vi "Router.vi"(8 "error in (no error)":errorcluster, 11 "Node Ptr":T1 format="%.0x") -> (0 "error out":errorcluster)   [LabVIEW 2016, in "PXImc Custom Device System Explorer.lvlib"]
uses:
  PXImc Custom Device System Explorer.lvlib
  <vilib>/NI Veristand/Custom Device API/Custom Device Item Ref.ctl
  Shared/Constants.vi
  <vilib>/NI Veristand/Custom Device API/Get Item Property (Variant).vi
  <vilib>/NI Veristand/Custom Device API/Set Item Property (Variant).vi
  <vilib>/NI VeriStand/Custom Device API/Custom Device API.lvlib
  Shared/PXImc Custom Device Shared.lvlib
panel:
  out "PXImc Resource Names":string[](array[string])
  in  "Connection Timeout (s)":dbl
  in  "Readers Buffer Size":u64
  in  "Configution Files Path":path
  in  "Load Configuration":bool
  in  "Header":cluster{"Section Name":string}={"Section Name"="Custom Device Item Settings"}
  in  "Description":string
  in  "Name":string
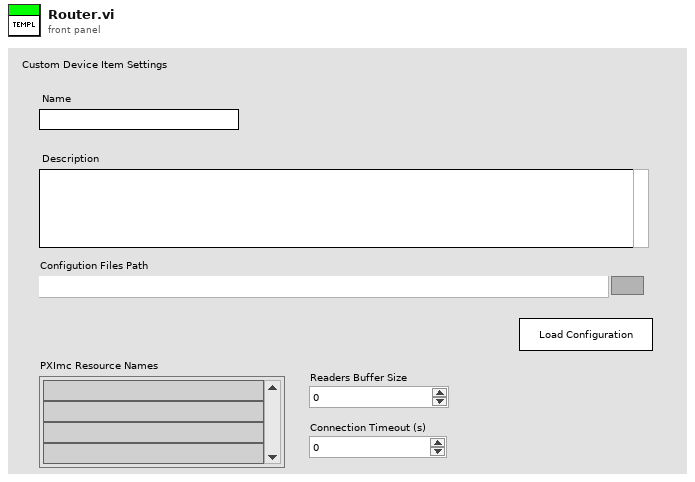
[diagram p1: front panel]
types:
  T1 = typedef "Custom Device API.lvlib/Custom Device Item Ref.ctl" = u64
  T2 = typedef "Custom Device API.lvlib/Custom Device Item Info.ctl" = cluster{"Name":string, "Is Channel":bool, "GUID":string, "Is Waveform":bool}
  T3 = typedef "PXImc Custom Device Shared.lvlib/Compiled.Settings.ctl" = cluster{"Target Type":T4, "Router Properties":T5, "Node Data":T10, "Configuration Folder Path":path}
  T4 = typedef "PXImc Router.lvlib/Target Type.ctl" = enum16{"Router", "Node"}
  T5 = typedef "PXImc Router.lvlib/Router - Configuration.ctl" = cluster{"Target Type":T4, "Master Table Ref":refnum<data-value>, "Master Table Size (Bytes)":u32, "Node Properties":T6[], "Router - PXImc Properties":T8}
  T6 = typedef "PXImc Router.lvlib/Node Block R-W Properties.ctl" = cluster{"Node ID":u32, "# Reading Blocks":u32, "Node Writing Block":T7, "Node Reading Blocks":T7[]}
  T7 = typedef "PXImc Router.lvlib/Block Properties.ctl" = cluster{"Offset":u32, "Size (Bytes)":u32}
  T8 = typedef "PXImc Router.lvlib/Router - PXImc Properties.ctl" = cluster{"PXImc Cards Properties":T9[], "Connection Timeout (s)":dbl, "Readers Buffer Size":u64}
  T9 = typedef "PXImc Router.lvlib/Router - PXImc Card Properties.ctl" = cluster{"PXImc Resource Name":string, "Reader - PXImc Session Ref":refnum<k21>, "Writer - PXImc Session Ref":refnum<k21>, "Reader Conn ID":u16, "Writer Conn ID":u16}
  T10 = typedef "PXImc Router.lvlib/Node Data.ctl" = cluster{"PXImc Parameters":T11, "Writer Data":T12, "Readers Data":T15}
  T11 = typedef "PXImc Router.lvlib/Node - PXImc Parameters.ctl" = cluster{"Resource Name":string, "Connection Timeout (s)":dbl, "Readers Buffer Size":u64, "Node PXImc Reader Conn Id":u16, "Node PXImc Writer Conn Id":u16, "Writer PXImc Session":refnum<k21>, "Reader PXImc Session":refnum<k21>}
  T12 = typedef "PXImc Router.lvlib/Node - Writer Data.ctl" = cluster{"Noder ID":u32, "Byte Buffer Ref":refnum<class "Byte Buffer.lvclass">, "Master Table Offest":u32, "Byte Buffer Size":u32, "Node Local Channels":T13[]}
  T13 = typedef "PXImc Router.lvlib/Node Ch Properties.ctl" = cluster{"Name":string, "Value":dbl, "Data Type":T14}
  T14 = typedef "PXImc Router.lvlib/Data Type.ctl" = enum16{"Boolean", "SGL", "DBL", "I8", "I16", "I32", "I64", "U8", "U16", "U32", "U64"}
  T15 = typedef "PXImc Router.lvlib/Node - Readers Data.ctl" = cluster{"Byte Buffer Ref":refnum<class "Byte Buffer.lvclass">, "Byte Buffer Size":u64, "Readers Data Array":T16[]}
  T16 = typedef "PXImc Router.lvlib/Node - Reader Data.ctl" = cluster{"Noder ID":u32, "Master Table Offest":u32, "Byte Buffer Size":u64, "Node Local Channels":T13[]}
  T17 = typedef "Custom Device API.lvlib/Custom Device Commands.ctl" = enum16{"Default", "Item renamed", "Shutdown", "Dynamic button pressed"}
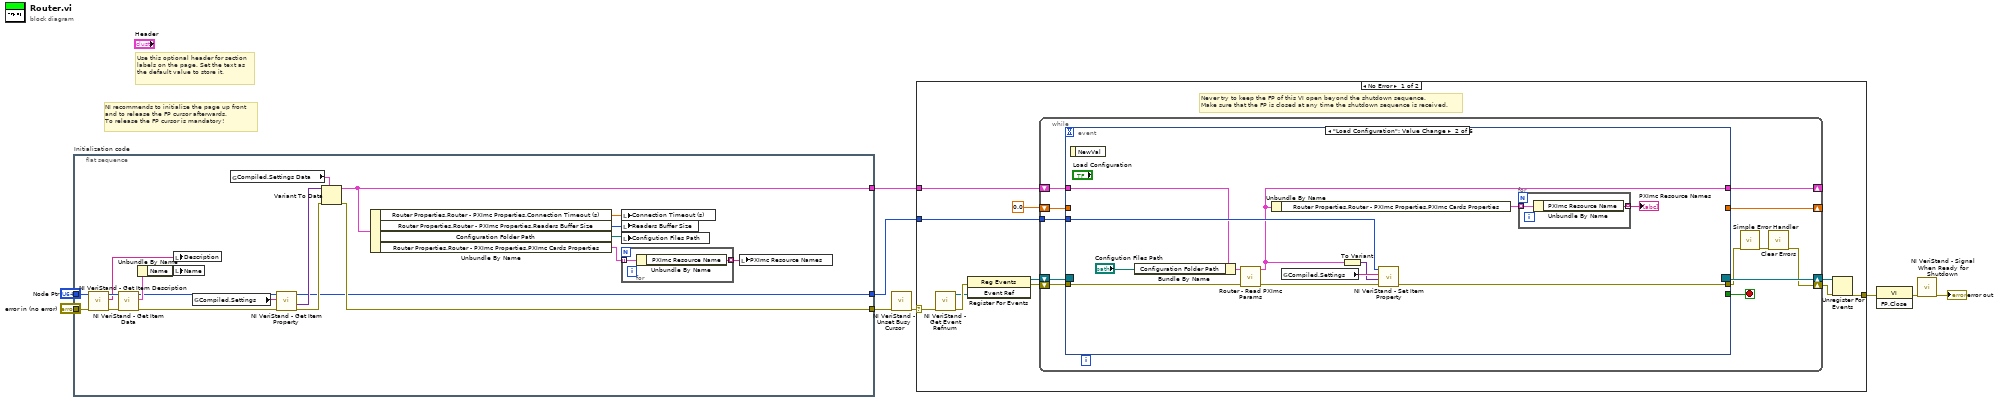
[diagram p0: block diagram]
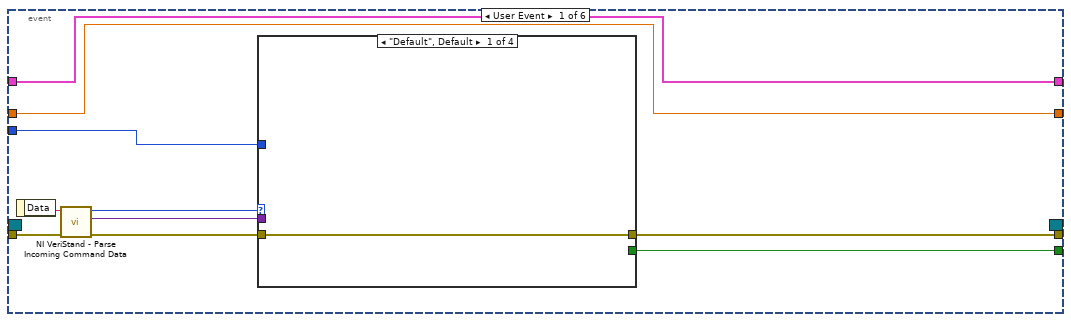
[diagram p2: hidden frame]
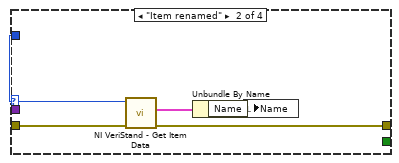
[diagram p3: hidden frame]
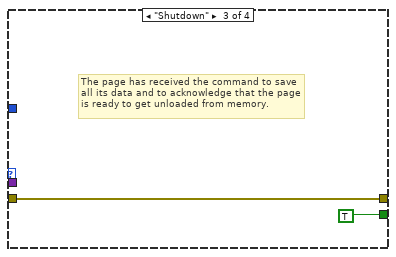
[diagram p4: hidden frame]
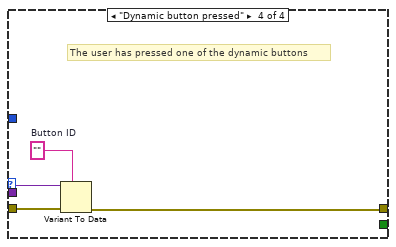
[diagram p5: hidden frame]
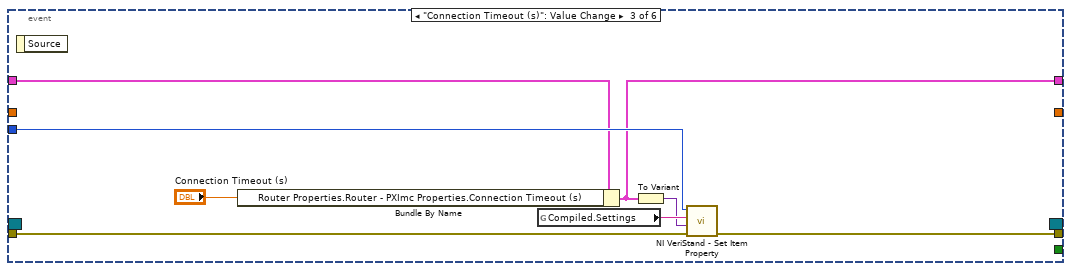
[diagram p6: hidden frame]
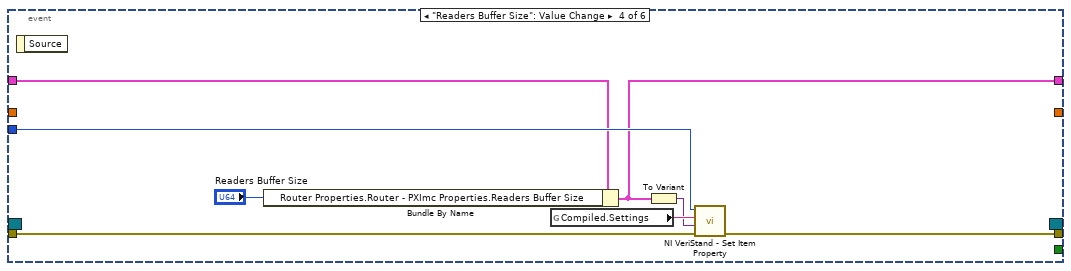
[diagram p7: hidden frame]
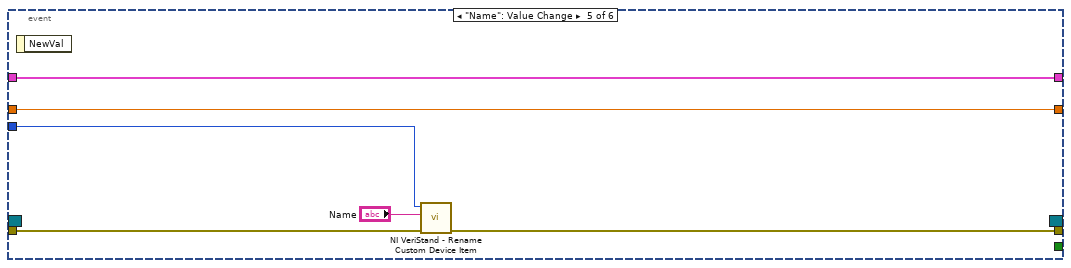
[diagram p8: hidden frame]
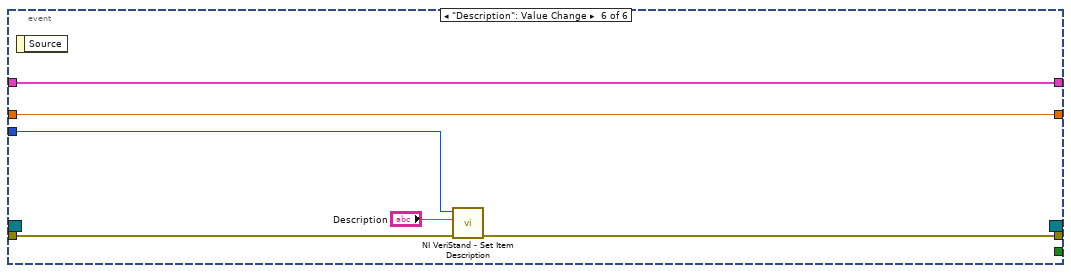
[diagram p9: hidden frame]
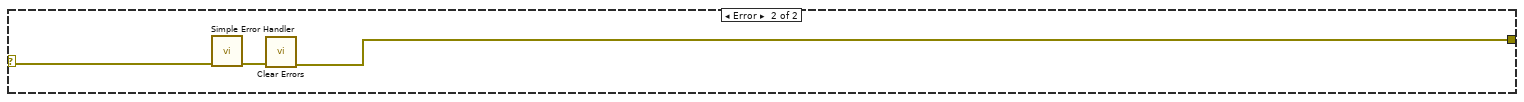
[diagram p10: hidden frame]
diagram:
  # "Use this optional header for section labels on the page. Set the text as the default value to store it."
  # "NI recommends to initialize the page up front\nand to release the FP cursor afterwards.\nTo release the FP cursor is mandatory!"
  n1 = flat-sequence "Initialization code" {
    tunnel: "error in (no error)" -> [w29]
    tunnel: "Node Ptr" -> [w28]
    tunnel: [w21] -> w5
    tunnel: [w14] -> w2
    tunnel: [w16] -> w1
    frame #0 {
      n2 = call <vilib>:"NI VeriStand - Get Item Description.vi"("error in (no error)"=w29, "Item Ref in"=w28) -> ("error out"=w26:errorcluster, "Description"=w27:string, "Item Ref out"=w30:T1)  [unwired: 7 out]
      n3 = call <vilib>:"NI VeriStand - Get Item Data.vi"("error in (no error)"=w26, "Item Ref in"=w30) -> ("error out"=w15:errorcluster, "Item Info"=w25:T2, "Item Ref out"=w17:T1)  [unwired: 7 out]
      n4 = Unbundle By Name(w25) -> ("Name"=w24:string)
      n5 = local write "Description"(w27) -> ()
      n6 = local write "Name"(w24) -> ()
      n7 = global read "Constants.vi" "Compiled.Settings"() -> (w20:string)
      n8 = global read "Constants.vi" "Compiled.Settings Data"() -> (w10:T3)
      n9 = call-poly <vilib>:"NI VeriStand - Get Item Property.vi"("error in (no error)"=w15, "Property Name"=w20, "Item Ref in"=w17) -> ("error out"=w22:errorcluster, "Value"=w23:variant, "Item Ref out"=w14:T1)  [unwired: 5 in, 1 out]
      n10 = Variant To Data(error in=w22, type=w10, Variant=w23) -> (data=w16:T3, error out=w21:errorcluster)
      n11 = Unbundle By Name(w16) -> ("Router Properties.Router - PXImc Properties.Connection Timeout (s)"=w19:dbl, "Router Properties.Router - PXImc Properties.Readers Buffer Size"=w18:u64, "Configuration Folder Path"=w13:path, "Router Properties.Router - PXImc Properties.PXImc Cards Properties"=w12:T9[])
      n12 = for {
        tunnel: w12 -> [w32] mode=indexing
        tunnel: [w31] -> w11 mode=indexing
        n13 = Unbundle By Name(w32) -> ("PXImc Resource Name"=w31:string)
      }
      n14 = local write "Connection Timeout (s)"(w19) -> ()
      n15 = local write "Readers Buffer Size"(w18) -> ()
      n16 = local write "Configution Files Path"(w13) -> ()
      n17 = local write "PXImc Resource Names"(w11) -> ()
    }
  }
  n18 = call <vilib>:"NI VeriStand - Unset Busy Cursor.vi"("error in (no error)"=w5) -> ("error out"=w4:errorcluster)  [unwired: 10 out]
  n19 = case shown="No Error" w4 {
    selector: w4 -> [w35 w122]
    tunnel: [w40 w120] -> w9
    tunnel: w2 -> [w36 _]
    tunnel: w1 -> [w33 _]
    frame No Error {
      # "Never try to keep the FP of this VI open beyond the shutdown sequence.\nMake sure that the FP is closed at any time the shutdown sequence is received."
      n20 = call <vilib>:"NI VeriStand - Get Event Refnum.vi"("error in (no error)"=w35) -> ("error out"=w43:errorcluster, "Event Ref"=w39:refnum<user-event>)  [unwired: 9 out]
      n21 = register-events(error in=w43, w39) -> (reference out=w37:refnum<event-registration>, error out=w38:errorcluster)  [unwired: 1 in]
      n22 = while {
        tunnel: w36 -> [w51]
        shift-right: [w48] -> w41
        shift-left: w38 -> [w54]
        shift-right: [w55] -> w42
        shift-left: w37 -> [w53]
        shift-right: [w46] -> _
        shift-left: 0.0 -> [w47]
        shift-right: [w44] -> _
        shift-left: w33 -> [w45]
        stop <- w52 stop-if-true
        n23 = event shown="[1] \"Load Configuration\": Value Change" {
          selector: w53 -> [_ _ _ _ _ _]
          dyn-events: [_ _ _ _ _ _] -> w55
          timeout: _ -> [_ _ _ _ _ _]
          tunnel: w54 -> [w65 w87 w98 w106 w113 w118]
          tunnel: [w61 _ _ _ _ _] -> w52
          tunnel: [w60 w89 w97 w105 w112 w117] -> w50
          tunnel: w51 -> [w59 w88 w99 w107 w111 w119]
          tunnel: w47 -> [w57 _ _ _ w109 w115]
          tunnel: [w57 _ _ _ w109 w115] -> w46
          tunnel: w45 -> [w56 w83 w94 w102 w108 w114]
          tunnel: [w56 w80 w93 w100 w108 w114] -> w44
          event User Event {
            n24 = event-data() -> ("Data"=w64:string)  [unwired: 1 out]
            n25 = call <vilib>:"NI VeriStand - Parse Incoming Command Data.vi"("error in (no error)"=w65, "Incoming data"=w64) -> ("error out"=w63:errorcluster, "Outgoing data"=w58:variant, "Action"=w62:T17)  [unwired: 7 out]
            n26 = case shown="\"Default\", Default" w62 {
              tunnel: w63 -> [w66 w71 w72 w77]
              tunnel: [_ _ TRUE _] -> w61
              tunnel: [w66 w68 w72 w74] -> w60
              tunnel: w59 -> [_ w70 _ _]
              tunnel: w58 -> [_ _ _ w76]
              frame "Default", Default {
              }
              frame "Item renamed" {
                n27 = call <vilib>:"NI VeriStand - Get Item Data.vi"("error in (no error)"=w71, "Item Ref in"=w70) -> ("error out"=w68:errorcluster, "Item Info"=w69:T2)  [unwired: 8 out]
                n28 = Unbundle By Name(w69) -> ("Name"=w67:string)
                n29 = local write "Name"(w67) -> ()
              }
              frame "Shutdown" {
                # "The page has received the command to save all its data and to acknowledge that the page is ready to get unloaded from memory."
              }
              frame "Dynamic button pressed" {
                w75 = ""  # Button ID
                # "The user has pressed one of the dynamic buttons"
                n30 = Variant To Data(error in=w77, type=w75, Variant=w76) -> (error out=w74:errorcluster)  [unwired: 1 out]
              }
            }
          }
          event "Load Configuration": Value Change {
            n31 = event-data() -> ()  [unwired: 2 out]
            n32 = Bundle By Name(cluster=w83, "Configuration Folder Path"="Configution Files Path") -> (w82:T3)
            n33 = call "Router - Read PXImc Params.vi"("error in (no error)"=w87, "Compiled.Settings In"=w82) -> ("error out"=w86:errorcluster, "Compiled.Settings Out"=w80:T3)  [unwired: 8 in]
            n34 = Unbundle By Name(w80) -> ("Router Properties.Router - PXImc Properties.PXImc Cards Properties"=w79:T9[])
            n35 = global read "Constants.vi" "Compiled.Settings"() -> (w85:string)
            n36 = To Variant(anything=w80) -> (Variant=w84:variant)
            n37 = call-poly <vilib>:"NI VeriStand - Set Item Property.vi"("error in (no error)"=w86, "Value"=w84, "Property Name"=w85, "Item Ref in"=w88) -> ("error out"=w89:errorcluster)  [unwired: 5 in, 2 out]
            n38 = for {
              tunnel: w79 -> [w91] mode=indexing
              tunnel: [w90] -> w78 mode=indexing
              n39 = Unbundle By Name(w91) -> ("PXImc Resource Name"=w90:string)
            }
            "PXImc Resource Names" <- w78
          }
          event "Connection Timeout (s)": Value Change {
            n40 = event-data() -> ()  [unwired: 2 out]
            n41 = Bundle By Name(cluster=w94, "Router Properties.Router - PXImc Properties.Connection Timeout (s)"="Connection Timeout (s)") -> (w93:T3)
            n42 = global read "Constants.vi" "Compiled.Settings"() -> (w96:string)
            n43 = To Variant(anything=w93) -> (Variant=w95:variant)
            n44 = call-poly <vilib>:"NI VeriStand - Set Item Property.vi"("error in (no error)"=w98, "Value"=w95, "Property Name"=w96, "Item Ref in"=w99) -> ("error out"=w97:errorcluster)  [unwired: 5 in, 2 out]
          }
          event "Readers Buffer Size": Value Change {
            n45 = event-data() -> ()  [unwired: 2 out]
            n46 = Bundle By Name(cluster=w102, "Router Properties.Router - PXImc Properties.Readers Buffer Size"="Readers Buffer Size") -> (w100:T3)
            n47 = global read "Constants.vi" "Compiled.Settings"() -> (w104:string)
            n48 = To Variant(anything=w100) -> (Variant=w103:variant)
            n49 = call-poly <vilib>:"NI VeriStand - Set Item Property.vi"("error in (no error)"=w106, "Value"=w103, "Property Name"=w104, "Item Ref in"=w107) -> ("error out"=w105:errorcluster)  [unwired: 5 in, 2 out]
          }
          event "Name": Value Change {
            n50 = event-data() -> ()  [unwired: 2 out]
            n51 = call <vilib>:"NI VeriStand - Rename Custom Device Item.vi"("error in (no error)"=w113, "New Name"="Name", "Item Ref in"=w111) -> ("error out"=w112:errorcluster)  [unwired: 1 in, 7 out]
          }
          event "Description": Value Change {
            n52 = event-data() -> ()  [unwired: 2 out]
            n53 = call <vilib>:"NI VeriStand - Set Item Description.vi"("error in (no error)"=w118, "Description"="Description", "Item Ref in"=w119) -> ("error out"=w117:errorcluster)  [unwired: 8 out]
          }
        }
        n54 = call <vilib>:"Simple Error Handler.vi"("error in (no error)"=w50) -> ("error out"=w49:errorcluster)  [unwired: 1 in, 7 out]
        n55 = call <vilib>:"Clear Errors.vi"("error in (no error)"=w49) -> ("error out"=w48:errorcluster)  [unwired: 1 in, 5 out]
      }
      n56 = Unregister For Events(event registration refnum=w42, error in=w41) -> (error out=w40:errorcluster)
    }
    frame Error {
      n57 = call <vilib>:"Simple Error Handler.vi"("error in (no error)"=w122) -> ("error out"=w121:errorcluster)  [unwired: 1 in, 7 out]
      n58 = call <vilib>:"Clear Errors.vi"("error in (no error)"=w121) -> ("error out"=w120:errorcluster)  [unwired: 1 in, 5 out]
    }
  }
  n59 = invoke class="VI" method="FP.Close"(error in=w9) -> (error out=w8:errorcluster)  [unwired: 2 in, 2 out]
  n60 = call <vilib>:"NI VeriStand - Signal When Ready for Shutdown.vi"("error in (no error)"=w8) -> ("error out"=→"error out":errorcluster)  [unwired: 10 out]
